vi "Number of Rows.vi"(8 "error in (no error)":errorcluster, 11 "PQ Result in":refnum<class "PQ Result.lvclass">) -> (0 "error out":errorcluster, 2 "Number of Rows":i32, 3 "PQ Result out":refnum<class "PQ Result.lvclass">)   [LabVIEW 2015, in "PQ Result.lvclass"]
uses:
  PQ Result.lvclass
  PQ Result.lvclass/PQ Result.ctl
  Connection/libpq.dll
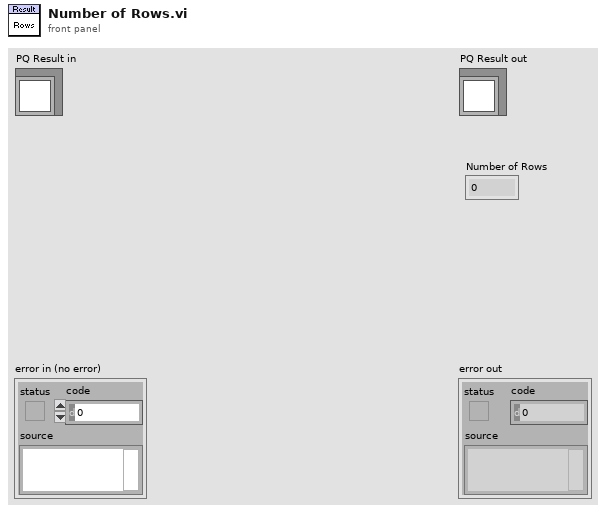
[diagram p1: front panel]
types:
  T1 = typedef "Result Status.ctl" = enum32{"PGRES_EMPTY_QUERY", "PGRES_COMMAND_OK", "PGRES_TUPLES_OK", "PGRES_COPY_OUT", "PGRES_COPY_IN", "PGRES_BAD_RESPONSE", "PGRES_NONFATAL_ERROR", "PGRES_FATAL_ERROR", "PGRES_COPY_BOTH", "PGRES_SINGLE_TUPLE"}
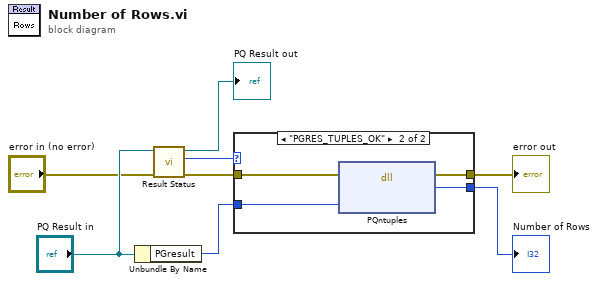
[diagram p0: block diagram]
diagram:
  n1 = Unbundle By Name("PQ Result in") -> ("PGresult"=w4:u32)
  n2 = call "Result Status.vi"("error in (no error)"="error in (no error)", "PQ Result in"="PQ Result in") -> ("error out"=w1:errorcluster, "Result Status"=w3:T1, "PQ Result out"=→"PQ Result out":refnum<class "PQ Result.lvclass">)  [unwired: 7 in]
  n3 = case shown="\"PGRES_TUPLES_OK\"" w3 {
    tunnel: [w9 w13] -> w8
    tunnel: [_ w12] -> w7
    tunnel: w1 -> [w9 w11]
    tunnel: w4 -> [_ w10]
    frame "PGRES_EMPTY_QUERY", Default {
    }
    frame "PGRES_TUPLES_OK" {
      n4 = dll-call lib="C:/PQ/Connection/libpq.dll" fn="PQntuples"(error in=w11, "PGresult"=w10) -> (error out=w13:errorcluster, "PQntuples"=w12:i32)  [unwired: 3 in, 1 out]
    }
  }
  "error out" <- w8
  "Number of Rows" <- w7
